vi "Theta, Phi angles Loop Iteration.vi"   [LabVIEW 2024]
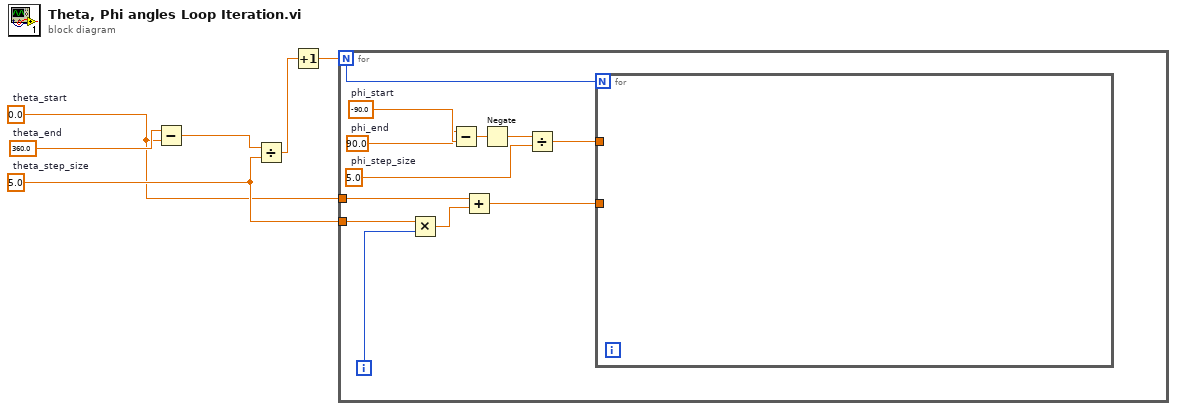
[diagram p0: block diagram]
diagram:
  w3 = 5.0  # theta_step_size
  w6 = 360.0  # theta_end
  w2 = 0.0  # theta_start
  n1 = Subtract(x=w6, y=w2) -> (x-y=w5:dbl)
  n2 = Divide(x=w5, y=w3) -> (x/y=w4:dbl)
  n3 = Increment(x=w4) -> (x+1=w1:dbl)
  n4 = for {
    N: w1 -> [w7]
    tunnel: w3 -> [w16]
    tunnel: w2 -> [w18]
    i -> [w15]
    w11 = 5.0  # phi_step_size
    w13 = 90.0  # phi_end
    w14 = -90.0  # phi_start
    n5 = Multiply(x=w16, y=w15) -> (x*y=w17:dbl)
    n6 = Subtract(x=w13, y=w14) -> (x-y=w12:dbl)
    n7 = Add(x=w18, y=w17) -> (x+y=w8:dbl)
    n8 = Negate(x=w12) -> (-x=w10:dbl)
    n9 = Divide(x=w10, y=w11) -> (x/y=w9:dbl)
    n10 = for {
      N: w7 -> [_]
      tunnel: w9 -> [_]
      tunnel: w8 -> [_]
    }
  }
